vi "(8) Encoder Version Set - Home Reference Attempt 2.vi"(0 "reference (in)":refnum<class "_Controller.lvclass">, 3 "Move":bool, 7 "error in (no error)":errorcluster) -> (20 "reference (out)":refnum<class "_Controller.lvclass">, 27 "error out":errorcluster)   [LabVIEW 2020]
uses:
  <instrlib>/Arcus Ethernet Driver 1.0.0/ArcusEthernetComm/classes/Controller/_Controller.lvclass
panel:
  out "Z Response":string
  out "Y Response":string
  out "X Response":string
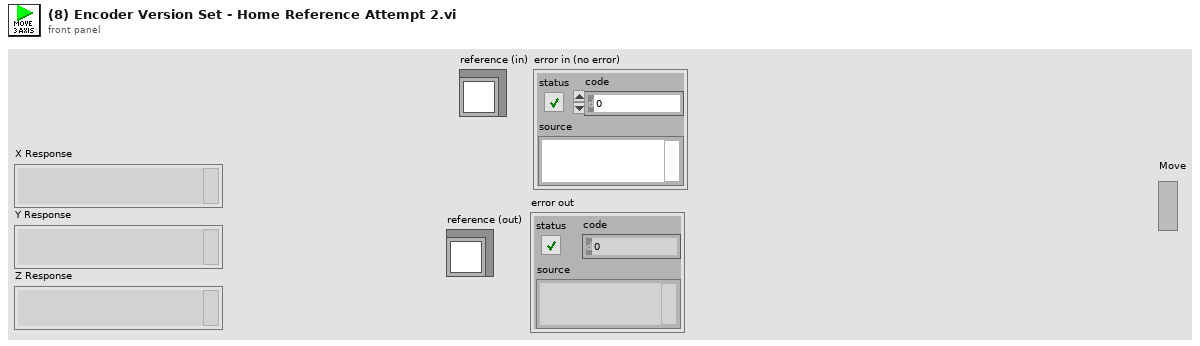
[diagram p1: front panel]
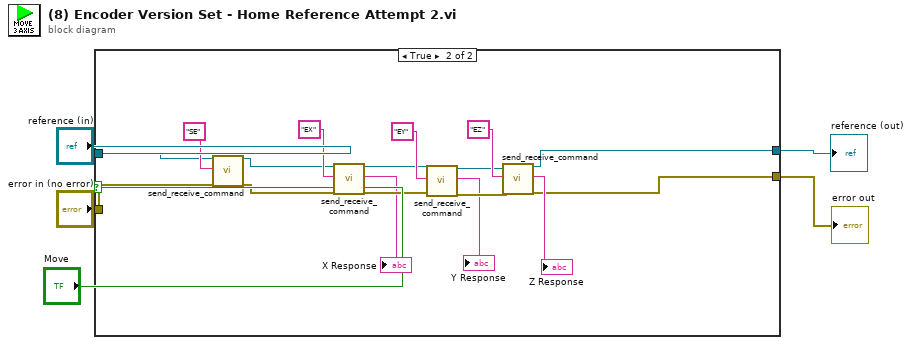
[diagram p0: block diagram]
diagram:
  n1 = case shown="True" "Move" {
    tunnel: "reference (in)" -> [w7 w22]
    tunnel: "error in (no error)" -> [w6 w23]
    tunnel: [w7 w9] -> w3
    tunnel: [w6 w8] -> w2
    frame False {
    }
    frame True {
      n2 = call <instrlib>:"send_receive_command.vi"("reference (in)"=w22, "ASCII Command (in)"="SE", "error in (no error)"=w23) -> ("reference (out)"=w11:refnum<class "_Controller.lvclass">, "error out"=w10:errorcluster)  [unwired: 12 in, 3 out]
      n3 = call <instrlib>:"send_receive_command.vi"("reference (in)"=w11, "ASCII Command (in)"="EX", "error in (no error)"=w10) -> ("reference (out)"=w19:refnum<class "_Controller.lvclass">, "response (out)"=→"X Response":string, "error out"=w18:errorcluster)  [unwired: 12 in, 2 out]
      n4 = call <instrlib>:"send_receive_command.vi"("reference (in)"=w19, "ASCII Command (in)"="EY", "error in (no error)"=w18) -> ("reference (out)"=w16:refnum<class "_Controller.lvclass">, "response (out)"=→"Y Response":string, "error out"=w15:errorcluster)  [unwired: 12 in, 2 out]
      n5 = call <instrlib>:"send_receive_command.vi"("reference (in)"=w16, "ASCII Command (in)"="EZ", "error in (no error)"=w15) -> ("reference (out)"=w9:refnum<class "_Controller.lvclass">, "response (out)"=→"Z Response":string, "error out"=w8:errorcluster)  [unwired: 12 in, 2 out]
    }
  }
  "reference (out)" <- w3
  "error out" <- w2
